vi "SinglePoint-AddResultChannels.vi"(8 "Error in":errorcluster, 11 "Custom Device ref":T1 format="%.0x") -> (0 "Error out":errorcluster, 3 "Custom Device ref out":T1 format="%.0x")   [LabVIEW 2014, in "Waveform-Processing-Custom-Device Shared.lvlib" / "SinglePoint.lvlib"]
uses:
  SinglePoint.lvlib
  <vilib>/NI Veristand/Custom Device API/Custom Device Item Ref.ctl
  <vilib>/NI Veristand/Custom Device API/Custom Device Channel.ctl
  <vilib>/NI Veristand/Custom Device API/Custom Device Channel Type.ctl
  NationalInstruments.VeriStand.SystemStorage
  Constants.vi
  <vilib>/NI Veristand/Custom Device API/Get Item Property (Dependent Node Pointer).vi
  <vilib>/NI Veristand/Custom Device API/Set Item Property (Dependent Node Pointer).vi
  <vilib>/NI Veristand/Custom Device API/Custom Device API.lvlib
  Waveform-Processing-Custom-Device Shared.lvlib
  System Explorer/Waveform-Processing-Custom-Device System Explorer.lvlib
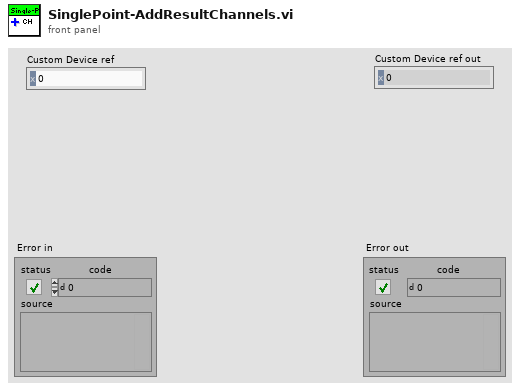
[diagram p1: front panel]
types:
  T1 = typedef "Custom Device API.lvlib/Custom Device Item Ref.ctl" = u64
  T2 = typedef "Custom Device API.lvlib/Custom Device Channel.ctl" = cluster{"Type":T3, "Units":string, "Default Value":dbl, "Faultable":bool, "Scalable":bool}
  T3 = typedef "Custom Device API.lvlib/Custom Device Channel Type.ctl" = enum16{"Input", "Output"}
  T4 = typedef "Custom Device API.lvlib/Custom Device Pointer.ctl" = refnum<k24>
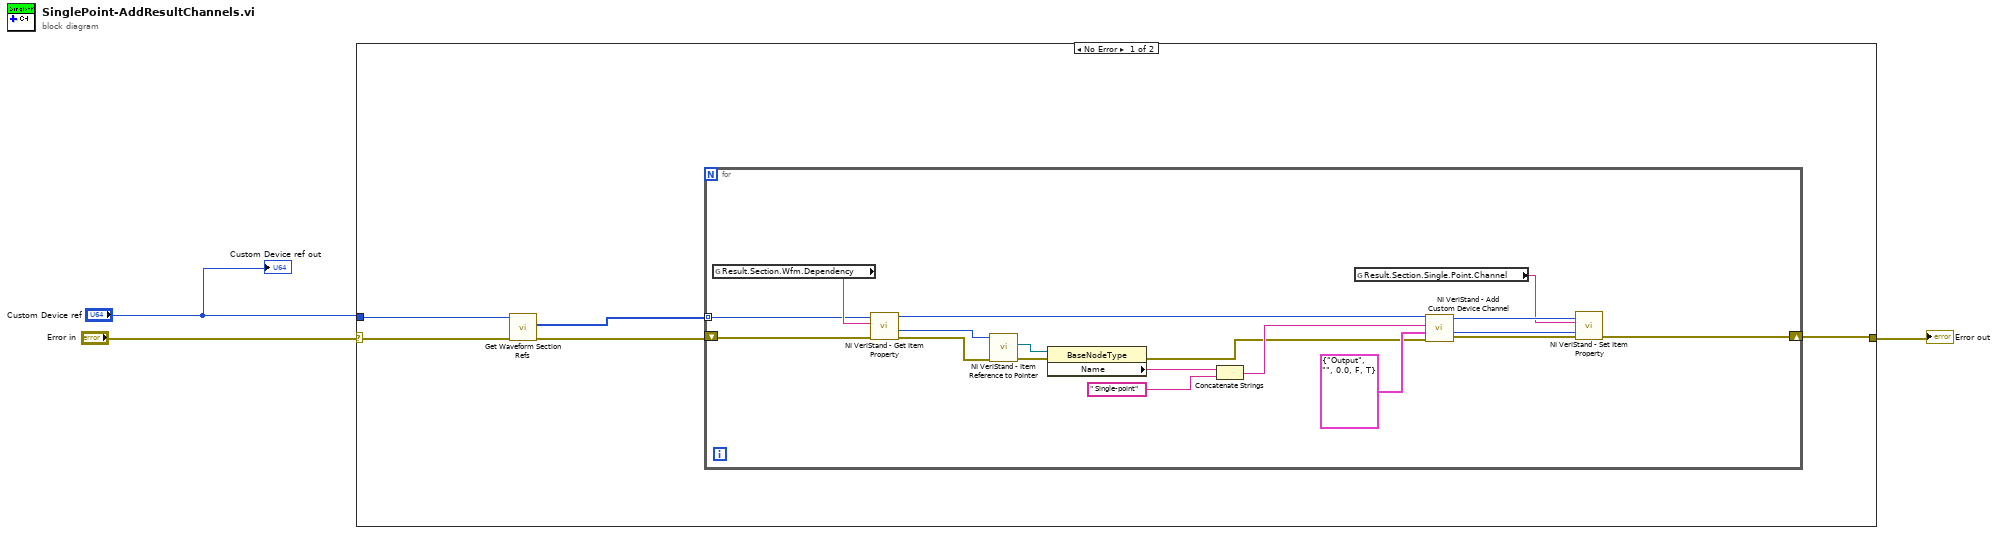
[diagram p0: block diagram]
diagram:
  n1 = case shown="No Error" "Error in" {
    selector: "Error in" -> [w8 w27]
    tunnel: "Custom Device ref" -> [w7 _]
    tunnel: [w4 w27] -> w2
    frame No Error {
      n2 = call "Get Waveform Section Refs.vi"("Error in"=w8, "Device Ref in"=w7) -> ("Error out"=w6:errorcluster, "Result Section Refs"=w5:T1[])  [unwired: 7 in, 1 out]
      n3 = for {
        tunnel: w5 -> [w17] mode=indexing
        shift-right: [w9] -> w4
        shift-left: w6 -> [w16]
        n4 = global read "Constants.vi" "Result.Section.Wfm.Dependency"() -> (w26:string)
        n5 = call-poly <vilib>:"NI VeriStand - Get Item Property.vi"("error in (no error)"=w16, "Property Name"=w26, "Item Ref in"=w17) -> ("error out"=w21:errorcluster, "Dependent Node Ref"=w22:T1, "Item Ref out"=w25:T1)  [unwired: 5 in, 1 out]
        n6 = call <vilib>:"NI VeriStand - Item Reference to Pointer.vi"("error in (no error)"=w21, "Item Ref in"=w22) -> ("error out"=w20:errorcluster, "Node Pointer"=w14:T4)  [unwired: 6 in, 2 out]
        n7 = property class="BaseNodeType"(reference=w14, error in=w20) -> (error out=w15:errorcluster, "Name"=w19:string)  [unwired: 1 out]
        n8 = Concatenate Strings(w19, " Single-point" ("Property Name")) -> (w24:string)
        n9 = global read "Constants.vi" "Result.Section.Single.Point.Channel"() -> (w10:string)
        n10 = call <vilib>:"NI VeriStand - Add Custom Device Channel.vi"("error in (no error)"=w15, "Channel"=T2 {"Type"=enum."Output", "Units"="", "Default Value"=0.0, "Faultable"=FALSE, "Scalable"=TRUE}, "Channel Name"=w24, "Parent Ref in"=w25) -> ("error out"=w13:errorcluster, "Channel Ref"=w11:T1, "Parent Ref out"=w12:T1)  [unwired: 4 in, 1 out]
        n11 = call-poly <vilib>:"NI VeriStand - Set Item Property.vi"("error in (no error)"=w13, "Dependent Node Ref"=w11, "Property Name"=w10, "Item Ref in"=w12) -> ("error out"=w9:errorcluster)  [unwired: 5 in, 2 out]
      }
    }
    frame Error {
    }
  }
  "Error out" <- w2
  "Custom Device ref out" <- "Custom Device ref"
